vi "IsConnected.vi"(8 "error in (no error)":errorcluster, 11 "QueueReader in":refnum<class "MultiQueueReader.lvclass">) -> (0 "error out":errorcluster, 2 "connected?":bool, 3 "QueueReader out":refnum<class "MultiQueueReader.lvclass">)   [LabVIEW 2013, in "MultiQueueReader.lvclass"]
doc: "Returns TRUE if the Readers connection is alive"
uses:
  MultiQueueReader.lvclass
  MultiQueueReader.lvclass/MultiQueueReader.ctl
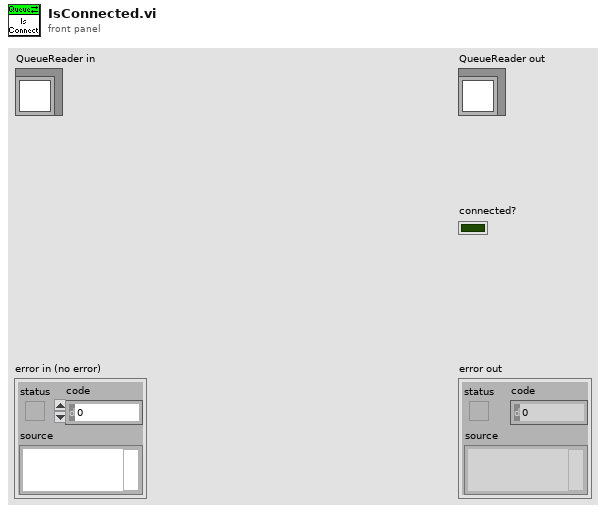
[diagram p1: front panel]
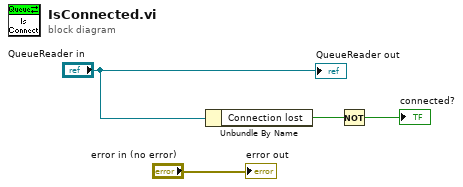
[diagram p0: block diagram]
diagram:
  n1 = Unbundle By Name("QueueReader in") -> ("Connection lost"=w2:bool)
  n2 = Not(x=w2) -> (.not. x?=→"connected?":bool)
  "error out" <- "error in (no error)"
  "QueueReader out" <- "QueueReader in"
